vi "exponential histogram model separate tau.vi"(3 "output control":T1, 4 "data":variant, 5 "X":dbl[](array[numeric]), 6 "a":dbl[](array[numeric])) -> (0 "error out":errorcluster, 1 "f'(X,a)":dbl[][](array[numeric]), 2 "f(X,a)":dbl[](array[numeric]))   [LabVIEW 2017]
doc: "Sum of three Gaussians, plus DC offset."
uses:
  <vilib>/gmath/NumericalOptimization/LM_output select.ctl
  <vilib>/gmath/NI_Gmath.lvlib
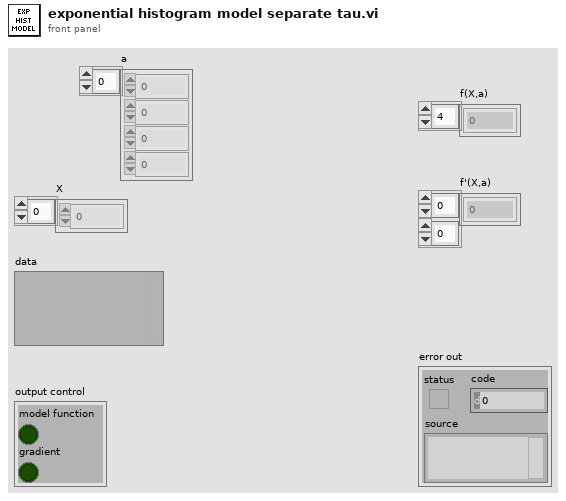
[diagram p1: front panel]
types:
  T1 = typedef "NI_Gmath.lvlib/LM_output select.ctl" = cluster{"model function":bool, "gradient":bool}
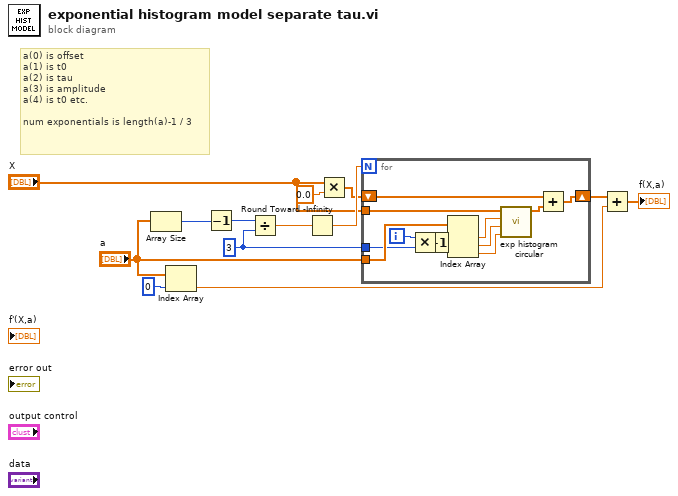
[diagram p0: block diagram]
diagram:
  w9 = 3 ("y")
  # "a(0) is offset\na(1) is t0\na(2) is tau\na(3) is amplitude\na(4) is t0 etc.\n\nnum exponentials is length(a)-1 / 3"
  n1 = Array Size(array="a") -> (size(s)=w13:i32)
  n2 = Index Array(array="a", index=0) -> (element=w2:dbl)
  n3 = Decrement(x=w13) -> (x-1=w12:i32)
  n4 = Divide(x=w12, y=w9) -> (x/y=w11:dbl)
  n5 = Round Toward -Infinity(1:w11) -> (0:w10:dbl)
  n6 = Multiply(x="X", y=0.0) -> (x*y=w6:dbl[])
  n7 = for {
    N: w10 -> [_]
    tunnel: "X" -> [w25]
    tunnel: "a" -> [w24]
    tunnel: w9 -> [w22]
    shift-right: [w15] -> w5
    shift-left: w6 -> [w16]
    i -> [w23]
    n8 = Multiply(x=w23, y=w22) -> (x*y=w21:i32)
    n9 = Increment(x=w21) -> (x+1=w14:i32)
    n10 = Index Array(array=w24, index #1=w14) -> (element #1=w20:dbl, element #2=w19:dbl, element #3=w18:dbl)  [unwired: 2 in]
    n11 = call "exp histogram circular.vi"("amplitude"=w18, "tau"=w19, "t0"=w20, "bin number"=w25) -> ("hist prediction"=w17:dbl[])  [unwired: 7 in]
    n12 = Add(x=w16, y=w17) -> (x+y=w15:dbl[])
  }
  n13 = Add(x=w5, y=w2) -> (x+y=→"f(X,a)":dbl[])
